vi "test Loopback Timestamp.vi"(8 "error in":errorcluster, 11 "TestCase in":refnum<class "Loopback.lvclass">) -> (0 "error out":errorcluster, 3 "TestCase out":refnum<class "Loopback.lvclass">)   [LabVIEW 2020, in "Loopback.lvclass"]
uses:
  Loopback.lvclass
  C:/dev/niveristand-custom-device-testing-tools/VeriStandTestCase/VeriStandTestCase.lvclass
  485b7c2b-8320-4722-9ec7-d01f27c65546.vi
  94b1695b-f377-4b7f-b0ef-3ed20e67d1fe.vi
  <vilib>/NI VeriStand/Execution/Workspace/NI VeriStand - Get Single Channel Value.vi
  <vilib>/NI VeriStand/Execution/Workspace/NI VeriStand - Get Multiple Channel Values.vi
  <vilib>/addons/_JKI Toolkits/VI Tester/TestCase.llb/TestCase.lvclass
  <vilib>/NI VeriStand/Execution/Workspace/NI_VS Workspace ExecutionAPI.lvlib
  C:/Program Files (x86)/National Instruments/LabVIEW 2020/vi.lib/addons/_JKI Toolkits/VI Tester/TestCase.llb/TestCase.lvclass
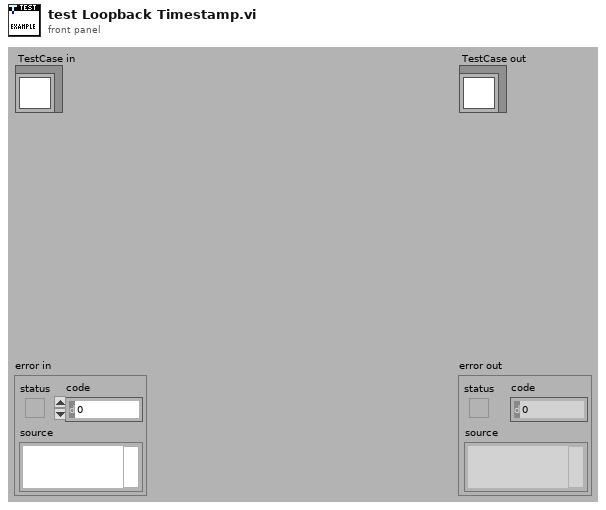
[diagram p1: front panel]
types:
  T1 = typedef "NI_VS Workspace ExecutionAPI.lvlib/WorkspaceAPI.ctl" = refnum<k24>
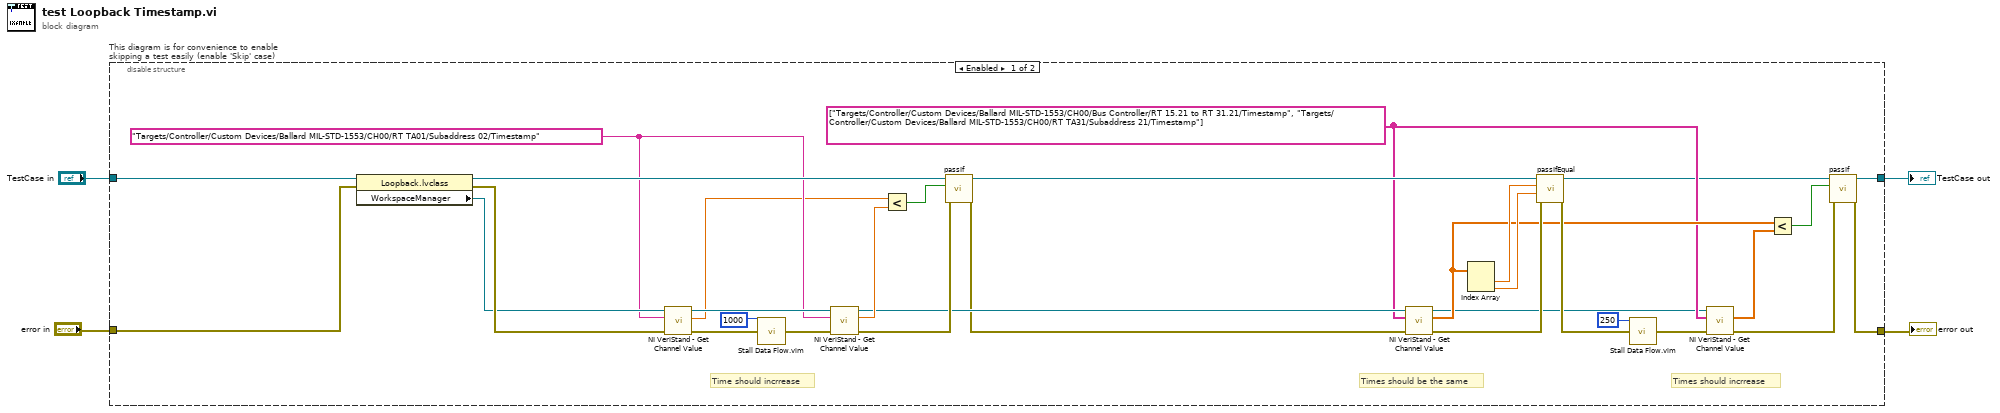
[diagram p0: block diagram]
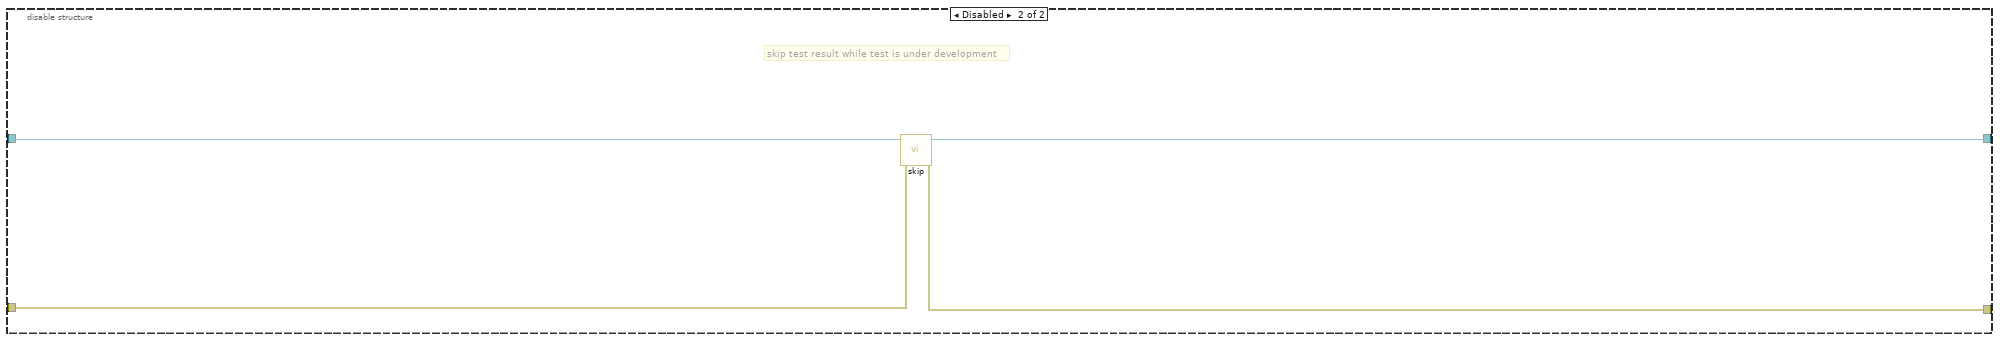
[diagram p2: hidden frame]
diagram:
  n1 = disable-structure "This diagram is for convenience to enable skipping a test easily (enable 'Skip' case)" shown="Enabled" {
    disable-tunnel: "TestCase in" -> [w28 w40]
    disable-tunnel: [w5 w39] -> w1
    disable-tunnel: [w11 w38] -> w3
    disable-tunnel: "error in" -> [w27 w37]
    frame Enabled {
      w8 = string[] ["Targets/Controller/Custom Devices/Ballard MIL-STD-1553/CH00/Bus Controller/RT 15.21 to RT 31.21/Timestamp", "Targets/Controller/Custom Devices/Ballard MIL-STD-1553/CH00/RT TA31/Subaddress 21/Timestamp"] ("Channels")
      w24 = "Targets/Controller/Custom Devices/Ballard MIL-STD-1553/CH00/RT TA01/Subaddress 02/Timestamp"
      # "Times should incrrease"
      # "Times should be the same"
      # "Time should incrrease"
      n2 = property class="Loopback.lvclass"(reference=w28, error in=w27) -> (reference out=w36:refnum<class "Loopback.lvclass">, error out=w31:errorcluster, "WorkspaceManager"=w29:T1)
      n3 = call-poly <vilib>:"NI VeriStand - Get Channel Value.vi"("error in (no error)"=w31, "Channel"=w24, "WorkspaceManager in"=w29) -> ("error out"=w33:errorcluster, "Value"=w23:dbl, "WorkspaceManager out"=w35:T1)  [unwired: 6 in]
      n4 = call "Stall Data Flow.vim"("value in"=w33, "milliseconds to wait"=u32 1000) -> ("value out"=w34:errorcluster)  [unwired: 1 out]
      n5 = call-poly <vilib>:"NI VeriStand - Get Channel Value.vi"("error in (no error)"=w34, "Channel"=w24, "WorkspaceManager in"=w35) -> ("error out"=w30:errorcluster, "Value"=w22:dbl, "WorkspaceManager out"=w20:T1)  [unwired: 6 in]
      n6 = Less?(x=w23, y=w22) -> (x < y?=w21:bool)
      n7 = call-dynamic "passIf.vi"("error in (no error)"=w30, "pass"=w21, "TestCase in"=w36) -> ("error out"=w15:errorcluster, "TestCase out"=w25:refnum<class "Loopback.lvclass">)  [unwired: 7 in]
      n8 = call-poly <vilib>:"NI VeriStand - Get Channel Value.vi"("error in (no error)"=w15, "Channels"=w8, "WorkspaceManager in"=w20) -> ("error out"=w26:errorcluster, "Values"=w10:dbl[], "WorkspaceManager out"=w7:T1)  [unwired: 6 in]
      n9 = Index Array(array=w10) -> (element #1=w19:dbl, element #2=w18:dbl)  [unwired: 2 in]
      n10 = call-dynamic "passIfEqual.vi"("error in (no error)"=w26, "y"=w18, "x"=w19, "TestCase in"=w25) -> ("error out"=w17:errorcluster, "TestCase out"=w6:refnum<class "Loopback.lvclass">)  [unwired: 6 in]
      n11 = call "Stall Data Flow.vim"("value in"=w17, "milliseconds to wait"=u32 250) -> ("value out"=w14:errorcluster)  [unwired: 1 out]
      n12 = call-poly <vilib>:"NI VeriStand - Get Channel Value.vi"("error in (no error)"=w14, "Channels"=w8, "WorkspaceManager in"=w7) -> ("error out"=w12:errorcluster, "Values"=w9:dbl[])  [unwired: 6 in, 1 out]
      n13 = Less?(x=w10, y=w9) -> (x < y?=w13:bool)
      n14 = call-dynamic "passIf.vi"("error in (no error)"=w12, "pass"=w13, "TestCase in"=w6) -> ("error out"=w11:errorcluster, "TestCase out"=w5:refnum<class "Loopback.lvclass">)  [unwired: 7 in]
    }
    frame Disabled {
      # "skip test result while test is under development"
      n15 = call <vilib>:"skip.vi"("error in (no error)"=w37, "TestCase in"=w40) -> ("error out"=w38:errorcluster, "TestCase out"=w39:refnum<class "Loopback.lvclass">)  [unwired: 8 in]
    }
  }
  "error out" <- w3
  "TestCase out" <- w1
